vi "rotate.vi"(0 "Angle":dbl, 3 "Rate":dbl) -> (7 "left speed":dbl, 8 "finished?":bool, 9 "right speed":dbl)   [LabVIEW 2014]
doc: "Rotates the robot for a certain number of degrees at a certain rate."
uses:
  global variables/robot_const.vi
  global variables/devrefs.vi
  <vilib>/addons/control/pid/pid.llb/PID Control Input Filter (DBL).vi
  <vilib>/addons/control/pid/NI_PID_pid.lvlib
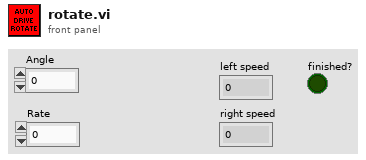
[diagram p1: front panel]
types:
  T1 = typedef "WPI_EncoderDevRef.ctl" = cluster{"DevStatus":errorcluster, "EncoderIndex":T2, "CounterIndex":T3, "DistancePerCount":dbl, "Decoding Type":T4}
  T2 = typedef "FPGA_EncoderIdx.ctl" = enum8{"Enc 0", "Enc 1", "Enc 2", "Enc 3", "Enc 4", "Enc 5", "Enc 6", "Enc 7", "Invalid"}
  T3 = typedef "FPGA_CounterCtrSystemIndex.ctl" = enum8{"Ctr 0", "Ctr 1", "Ctr 2", "Ctr 3", "Ctr 4", "Ctr 5", "Ctr 6", "Ctr 7", "Invalid"}
  T4 = typedef "WPI_EncoderType.ctl" = enum16{"1x", "2x", "4x"}
  T5 = typedef "subStates.ctl" = enum16{"null", "wait", "driver control", "auto", "manual override", "hold position", "rotate", "test", "end"}
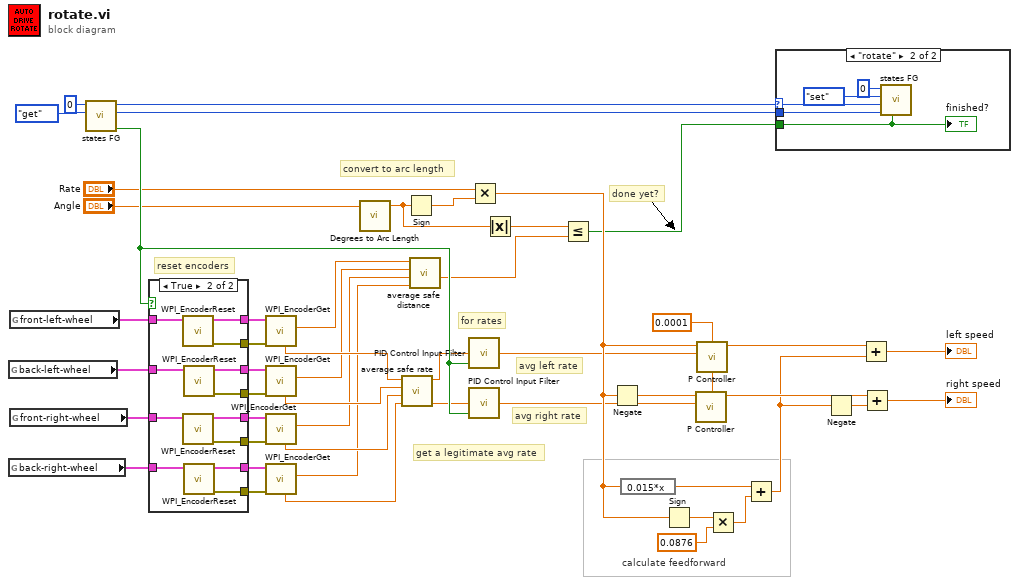
[diagram p0: block diagram]
diagram:
  w25 = 0.0001 ("proportional gain (Kc)")
  # "get a legitimate avg rate"
  # "convert to arc length"
  # "for rates"
  # "avg right rate"
  # "avg left rate"
  # "reset encoders"
  # "calculate feedforward"
  # "done yet?"
  n1 = global read "devrefs.vi" "back-left-wheel"() -> (w21:T1)
  n2 = global read "devrefs.vi" "back-right-wheel"() -> (w15:T1)
  n3 = global read "devrefs.vi" "front-left-wheel"() -> (w22:T1)
  n4 = global read "devrefs.vi" "front-right-wheel"() -> (w16:T1)
  n5 = call "states FG.vi"("menu (get)"=enum16{"set", "get"}."get", "Loop ID"=0) -> ("first call?"=w39:bool, "state # out"=w24:i32, "subState out"=w27:T5)  [unwired: 6 in, 1 out]
  n6 = case shown="True" w39 {
    tunnel: [_ w65] -> w45
    tunnel: [w50 w64] -> w44
    tunnel: [w51 w63] -> w43
    tunnel: [_ w62] -> w42
    tunnel: w22 -> [w50 w61]
    tunnel: w21 -> [w51 w60]
    tunnel: [_ w56] -> w17
    tunnel: [w52 w57] -> w18
    tunnel: [w53 w58] -> w19
    tunnel: [_ w59] -> w20
    tunnel: w16 -> [w52 w55]
    tunnel: w15 -> [w53 w54]
    frame False {
    }
    frame True {
      n7 = call <vilib>:"WPI_EncoderReset.vi"("EncoderDevRef"=w61) -> ("error out"=w65:errorcluster, "EncoderDevRef"=w64:T1)  [unwired: 9 in]
      n8 = call <vilib>:"WPI_EncoderReset.vi"("EncoderDevRef"=w55) -> ("error out"=w56:errorcluster, "EncoderDevRef"=w57:T1)  [unwired: 9 in]
      n9 = call <vilib>:"WPI_EncoderReset.vi"("EncoderDevRef"=w60) -> ("error out"=w62:errorcluster, "EncoderDevRef"=w63:T1)  [unwired: 9 in]
      n10 = call <vilib>:"WPI_EncoderReset.vi"("EncoderDevRef"=w54) -> ("error out"=w59:errorcluster, "EncoderDevRef"=w58:T1)  [unwired: 9 in]
    }
  }
  n11 = call <vilib>:"WPI_EncoderGet.vi"("error in (no error)"=w45, "EncoderDevRef"=w44) -> ("Distance"=w2:dbl, "Rate"=w11:dbl)  [unwired: 4 in, 4 out]
  n12 = call <vilib>:"WPI_EncoderGet.vi"("error in (no error)"=w42, "EncoderDevRef"=w43) -> ("Distance"=w3:dbl, "Rate"=w10:dbl)  [unwired: 4 in, 4 out]
  n13 = call <vilib>:"WPI_EncoderGet.vi"("error in (no error)"=w17, "EncoderDevRef"=w18) -> ("Distance"=w4:dbl, "Rate"=w9:dbl)  [unwired: 4 in, 4 out]
  n14 = call <vilib>:"WPI_EncoderGet.vi"("error in (no error)"=w20, "EncoderDevRef"=w19) -> ("Distance"=w5:dbl, "Rate"=w8:dbl)  [unwired: 4 in, 4 out]
  n15 = call "Degrees to Arc Length.vi"("Angle"="Angle") -> ("Arc Length (inches)"=w23:dbl)  [unwired: 4 in]
  n16 = call "average safe rate.vi"("Back Right"=w8, "Front Right"=w9, "Back Left"=w10, "Front Left"=w11) -> ("Right Average Rate"=w6:dbl, "Left Average Rate"=w7:dbl)  [unwired: 6 in]
  n17 = Sign(1:w23) -> (0:w37:dbl)
  n18 = call "average safe distance.vi"("Back Right"=w5, "Front Right"=w4, "Back Left"=w3, "Front Left"=w2) -> ("Average Absolute Distance"=w1:dbl)  [unwired: 2 in, 3 out]
  n19 = call-poly <vilib>:"PID Control Input Filter.vi"("reinitialize? (F)"=w39, "input"=w7) -> ("output"=w13:dbl)  [unwired: 3 in]
  n20 = call-poly <vilib>:"PID Control Input Filter.vi"("reinitialize? (F)"=w39, "input"=w6) -> ("output"=w12:dbl)  [unwired: 3 in]
  n21 = Multiply(x="Rate", y=w37) -> (x*y=w33:dbl)
  n22 = Absolute Value(x=w23) -> (abs(x)=w28:dbl)
  n23 = Less Or Equal?(x=w28, y=w1) -> (x <= y?=w14:bool)
  n24 = Negate(x=w33) -> (-x=w36:dbl)
  n25 = expression code="0.015*x"(w33) -> (w31:dbl)
  n26 = Sign(1:w33) -> (0:w35:dbl)
  n27 = call "P Controller.vi"("Kp"=w25, "Setpoint"=w36, "Process Variable"=w12) -> ("Output"=w49:dbl)  [unwired: 5 in]
  n28 = call "P Controller.vi"("Kp"=w25, "Setpoint"=w33, "Process Variable"=w13) -> ("Output"=w48:dbl)  [unwired: 5 in]
  n29 = Multiply(x=w35, y=0.0876) -> (x*y=w32:dbl)
  n30 = Add(x=w31, y=w32) -> (x+y=w29:dbl)
  n31 = case shown="\"rotate\"" w27 {
    selector: w27 -> [_ w66]
    tunnel: w14 -> [_ w69]
    tunnel: w24 -> [_ w67]
    frame "null", Default {
    }
    frame "rotate" {
      n32 = call "states FG.vi"("exit in"=w69, "state # in"=w67, "subState in"=w66, "menu (get)"=enum16{"set", "get"}."set", "Loop ID"=0) -> ()  [unwired: 3 in, 4 out]
      "finished?" <- w69
    }
  }
  n33 = Negate(x=w29) -> (-x=w30:dbl)
  n34 = Add(x=w48, y=w29) -> (x+y=→"left speed":dbl)
  n35 = Add(x=w49, y=w30) -> (x+y=→"right speed":dbl)
